vi "runtime io test.vi"() -> ()   [LabVIEW 2013, in "Shared Library Module tests.lvlib"]
doc: "Platypus Framework 1.0.1.60\nNI Systems Engineering - National Instruments"
uses:
  Shared Library Module tests.lvlib
  <vilib>/NI/Tag Bus Module Framework/channel/channel classification.ctl
  execution/Shared Library Module runtime.lvclass
  configuration/Shared Library Module configuration.lvclass
  <vilib>/NI/Tag Bus/tag/tag descriptor.lvclass/tag descriptor.ctl
  <vilib>/NI/Tag Bus/table/data polymorphs/write one/write Double.vi
  <vilib>/NI/Tag Bus/table/data polymorphs/read one/read Double.vi
  <vilib>/NI/Tag Bus/tag/read tag name.vi
  <vilib>/NI/Tag Bus/tag/read data type.vi
  <vilib>/NI/Tag Bus Module Framework/channel/TBM channel.lvclass
  <vilib>/NI/Tag Bus Module Framework/root configuration/TBM configuration.lvclass
  <vilib>/NI/Tag Bus/dictionary/data dictionary.lvclass
  <vilib>/NI/Tag Bus/table/data table.lvlib
panel:
  out "inputs changed?":bool
  out "no error":errorcluster
  # "This is expected to remain false until you write code for input"
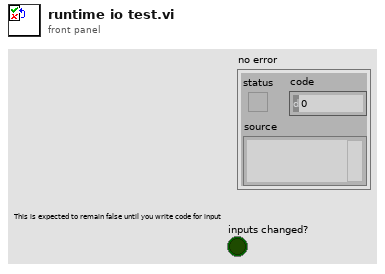
[diagram p1: front panel]
types:
  T1 = typedef "TBM channel.lvclass/channel classification.ctl" = enum16{"input data", "output data", "processing parameter", "processing result"}
  T2 = typedef "tag bus.lvlib/tag descriptor.lvclass/Data Type.ctl" = enum16{"Double", "Single", "I64", "I32", "I16", "I8", "U64", "U32", "U16", "U8", "Boolean", "String", "Array of Double", "Array of Single", "Array of I64", "Array of I32", "Array of I16", "Array of I8", "Array of U64", "Array of U32", "Array of U16", "Array of U8", "Array of Boolean", "Array of String"}
  T3 = typedef "TBM channel.lvclass/data tables.ctl" = cluster{"input data":T4, "processing parameter":T4, "processing result":T4, "output data":T4}
  T4 = typedef "tag bus.lvlib/dictionary table pair.ctl" = cluster{"data dictionary":refnum<class "data dictionary.lvclass">, "data table":T5}
  T5 = typedef "tag bus.lvlib/data table.lvlib/data table.ctl" = cluster{"Double":dbl[], "Single":sgl[], "I64":i64[], "I32":i32[], "I16":i16[], "I8":i8[], "U64":u64[], "U32":u32[], "U16":u16[], "U8":u8[], "Boolean":bool[], "String":string[], "Array of Double":cluster{"DBL Array":dbl[]}[], "Array of Single":cluster{"SGL Array":sgl[]}[], "Array of I64":cluster{"I64 Array":i64[]}[], "Array of I32":cluster{"I32 Array":i32[]}[], "Array of I16":cluster{"I16 Array":i16[]}[], "Array of I8":cluster{"I8 Array":i8[]}[], "Array of U64":cluster{"U64 Array":u64[]}[], "Array of U32":cluster{"U32 Array":u32[]}[], "Array of U16":cluster{"U16 Array":u16[]}[], "Array of U8":cluster{"U8 Array":u8[]}[], "Array of Boolean":cluster{"Boolean Array":bool[]}[], "Array of String":cluster{"String Array":string[]}[]}
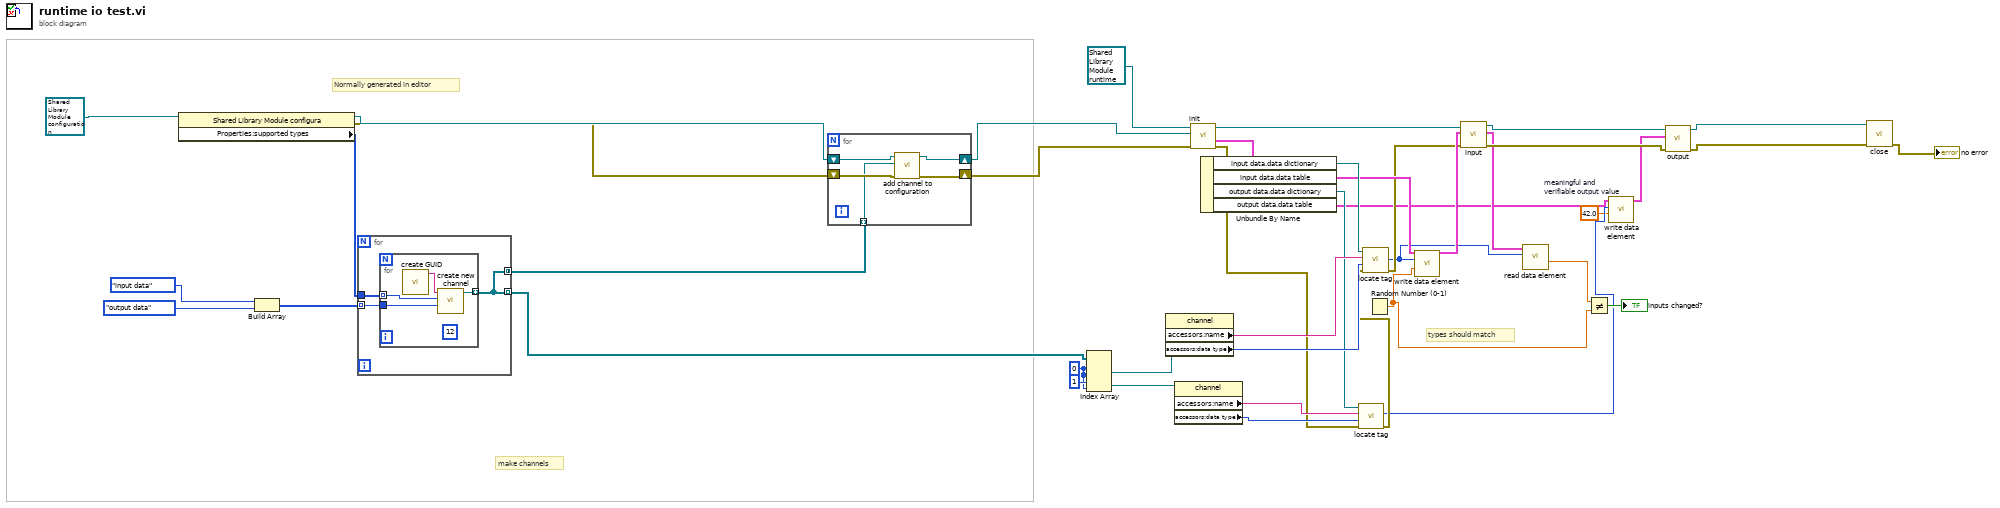
[diagram p0: block diagram]
diagram:
  w8 = 42.0  # meaningful and verifiable output value
  w37 = 0 ("index (row)")
  # "types should match"
  # "Normally generated in editor"
  # "make channels"
  n1 = property class="Shared Library Module configura"(reference=refnum<class "Shared Library Module configuration.lvclass"> refnum ("tag bus configurable plugin module configuration")) -> (reference out=w5:refnum<class "Shared Library Module configuration.lvclass">, error out=w2:errorcluster, "Properties:supported types"=w40:T2[])  [unwired: 1 in]
  n2 = Build Array(channel_classification."input data" ("channel classification"), channel_classification."output data" ("channel classification")) -> (w41:T1[])
  n3 = for {
    tunnel: w41 -> [w46] mode=indexing
    tunnel: [w44] -> w39 mode=indexing
    tunnel: w40 -> [w45]
    tunnel: [w44] -> w3 mode=concatenating
    n4 = for {
      tunnel: w46 -> [w49]
      tunnel: [w50] -> w44 mode=indexing
      tunnel: w45 -> [w48] mode=indexing
      (unwired) 12
      n5 = call <vilib>:"create GUID.vi"() -> ("uuid"=w47:string)  [unwired: 11 in]
      n6 = call <vilib>:"create new channel.vi"("channel classification"=w49, "data type"=w48, "channel name"=w47) -> ("channel"=w50:refnum<class "TBM channel.lvclass">)  [unwired: 8 in]
    }
  }
  n7 = for {
    shift-right: [w54] -> w4
    shift-left: w5 -> [w55]
    shift-right: [w53] -> w1
    shift-left: w2 -> [w52]
    tunnel: w3 -> [w51] mode=indexing
    n8 = call "add channel to configuration.vi"("error in"=w52, "TBM channel in"=w51, "Shared Library Module configuration in"=w55) -> ("error out"=w53:errorcluster, "Shared Library Module configuration out"=w54:refnum<class "Shared Library Module configuration.lvclass">)  [unwired: 7 in]
  }
  n9 = Index Array(array=w39, index (row) #1=w37, index (col) #1=w37, index (row) #2=1 ("index (row)"), index (col) #2=w37) -> (element #1=w28:refnum<class "TBM channel.lvclass">, element #2=w17:refnum<class "TBM channel.lvclass">)
  n10 = property class="channel"(reference=w28) -> ("accessors:name"=w26:string, "accessors:data type"=w27:T2)  [unwired: 1 in, 2 out]
  n11 = property class="channel"(reference=w17) -> ("accessors:name"=w15:string, "accessors:data type"=w14:T2)  [unwired: 1 in, 2 out]
  n12 = call-dynamic "init.vi"("error in"=w1, "TBM module configuration in"=w4, "Shared Library Module runtime in"=refnum<class "Shared Library Module runtime.lvclass"> refnum ("tag bus configurable plugin module")) -> ("error out"=w13:errorcluster, "data allocations"=w30:T3, "Shared Library Module runtime out"=w31:refnum<class "Shared Library Module runtime.lvclass">)  [unwired: 5 in, 1 out]
  n13 = Unbundle By Name(w30) -> ("input data.data dictionary"=w29:refnum<class "data dictionary.lvclass">, "input data.data table"=w25:T5, "output data.data dictionary"=w16:refnum<class "data dictionary.lvclass">, "output data.data table"=w11:T5)
  n14 = call <vilib>:"locate tag.vi"("error in"=w13, "data type"=w14, "name"=w15, "data dictionary in"=w16) -> ("error out"=w12:errorcluster, "index"=w9:i32)  [unwired: 5 in, 1 out]
  n15 = call <vilib>:"locate tag.vi"("error in"=w12, "data type"=w27, "name"=w26, "data dictionary in"=w29) -> ("error out"=w23:errorcluster, "index"=w21:i32)  [unwired: 5 in, 1 out]
  n16 = Random Number (0-1)() -> (number: 0 to 1=w20:dbl)
  n17 = call-poly <vilib>:"write data element.vi"("value"=w20, "index"=w21, "data table in"=w25) -> ("data table out"=w24:T5)  [unwired: 8 in]
  n18 = call-dynamic "input.vi"("error in"=w23, "data table in"=w24, "Shared Library Module runtime in"=w31) -> ("error out"=w32:errorcluster, "data table out"=w22:T5, "Shared Library Module runtime out"=w33:refnum<class "Shared Library Module runtime.lvclass">)  [unwired: 6 in]
  n19 = call-poly <vilib>:"read data element.vi"("index"=w21, "data table in"=w22) -> ("value"=w19:dbl)  [unwired: 8 in, 1 out]
  n20 = Not Equal?(x=w19, y=w20) -> (x != y?=→"inputs changed?":bool)
  n21 = call-poly <vilib>:"write data element.vi"("value"=w8, "index"=w9, "data table in"=w11) -> ("data table out"=w10:T5)  [unwired: 8 in]
  n22 = call-dynamic "output.vi"("error in"=w32, "data table in"=w10, "Shared Library Module runtime in"=w33) -> ("error out"=w34:errorcluster, "Shared Library Module runtime out"=w35:refnum<class "Shared Library Module runtime.lvclass">)  [unwired: 6 in, 1 out]
  n23 = call-dynamic "close.vi"("error in"=w34, "Shared Library Module runtime in"=w35) -> ("error out"=→"no error":errorcluster)  [unwired: 9 in]
